vi "Utilization.vi"() -> ()   [LabVIEW 2019]
uses:
  <vilib>/Skyline/AssetManagement/Start Utilization (Single).vi
  Asset/Asset.lvclass
  <vilib>/Skyline/AssetManagement/NI SystemLink Asset Utilization.lvclass
panel:
  in  "stop":bool
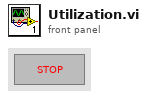
[diagram p1: front panel]
types:
  T1 = enum16{"BuiltInSystem", "PciPxi", "Usb", "Gpib", "Vxi", "Serial", "TcpIp", "cRio", "Scxi", "cDaq", "SwitchBlock", "Scc", "FireWire", "Accessory", "Can", "SwitchBlockDevice"}
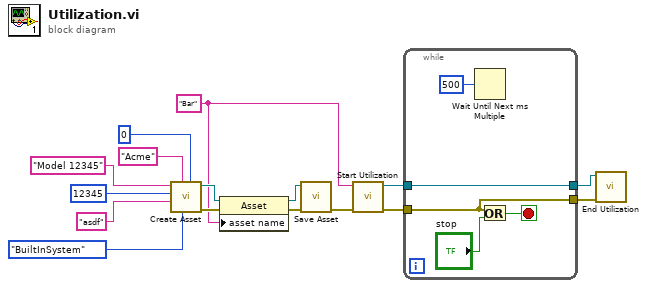
[diagram p0: block diagram]
diagram:
  w1 = "Bar" ("asset name")
  n1 = call "Create Asset.vi"("Vendor Number"=u32 0, "Bus Type"=T1."BuiltInSystem", "Vendor Name"="Acme", "Serial Number"="asdf", "Model Number"=u32 12345, "Model Name"="Model 12345") -> ("Error Out"=w5:errorcluster, "Asset"=w2:refnum<class "Asset.lvclass">)  [unwired: 4 in]
  n2 = property class="Asset"(reference=w2, error in=w5, "asset name"=w1) -> (reference out=w3:refnum<class "Asset.lvclass">, error out=w4:errorcluster)
  n3 = call "Save Asset.vi"("Error In"=w4, "Asset"=w3) -> ("Error Out"=w8:errorcluster)  [unwired: 9 in]
  n4 = call-poly <vilib>:"Start Utilization.vi"("error in (no error)"=w8, "asset name"=w1) -> ("error out"=w15:errorcluster, "asset utilization"=w16:refnum<class "NI SystemLink Asset Utilization.lvclass">)  [unwired: 8 in]
  n5 = while {
    tunnel: [w20] -> w13
    tunnel: w16 -> [w20]
    tunnel: w15 -> [w19]
    tunnel: [w19] -> w14
    stop <- w17 stop-if-true
    n6 = Wait Until Next ms Multiple(millisecond multiple=u32 500) -> ()  [unwired: 1 out]
    n7 = Or(x=w19, y="stop") -> (x .or. y?=w17:bool)
  }
  n8 = call <vilib>:"End Utilization.vi"("error in (no error)"=w14, "asset utilization"=w13) -> ()  [unwired: 9 in, 1 out]
